vi "Consumer.vi"(8 "error in (no error)":errorcluster, 9 "Data":variant, 10 "Case ID":string, 11 "uService Template in":refnum<class "DAQ Manager.lvclass">) -> (0 "error out":errorcluster, 3 "uService Template out":refnum<class "DAQ Manager.lvclass">)   [LabVIEW 2020, in "TALOS.lvlib" / "DAQ Manager.lvlib" / "DAQ Manager.lvclass"]
uses:
  DAQ Manager.lvclass
  C:/LabVIEW Code/TALOS/talos/Father of all uServices/Father of all uServices/Father of all uServices.lvclass
  DAQ Manager Consumer Case Selector.ctl
  Father of all uServices/Father of all uServices/Father of all uServices.lvclass/Father of all uServices.ctl
  Ancestor/Ancestor/Ancestor.lvclass/Ancestor.ctl
  Guardian/Guardian/Requests.ctl
  Guardian/Guardian Messages/Requests from uServices Msg/Requests from uServices Msg.lvclass/Requests from uServices Msg.ctl
  Guardian/Guardian Messages/Message to uService Msg/Message to uService Msg.lvclass/Message to uService Msg.ctl
  Interfaces/DAQ Control/Metadata.ctl
  Guardian/Guardian Messages/Requests from uServices Msg/Send Requests from uServices.vi
  Support VIs/Generate Error.vi
  Father of all uServices/Father of all uServices/Children Methods/Message to uService.vi
  FGV/Error Memory/Get Error Description.vi
  Support VIs/Get PC name.vi
  Ancestor/Ancestor/Read ID.vi
  Support VIs/Get Class Name.vi
  <vilib>/Utility/error.llb/Clear Errors.vi
  Guardian/Guardian Messages/Message to uService Msg/Send Message to uService.vi
  FGV/Error Memory/Error Memory Core.vi
  <vilib>/AdvancedString/Delimited String to 1D String Array.vi
  Support VIs/Circus Root Path.vi
  FGV/Error Memory/Error Crt Lvl checker.vi
  FGV/Error Memory/Error Memory Core.vi/40c8088d-b597-4017-91af-faa98e00292e.vi
  FGV/Error Memory/Error Memory Core.vi/d4a3ab98-063c-4e44-b43d-fbdcfe6c2be2.vi
  Father of all uServices/Father of all uServices/Father of all uServices.lvclass
  C:/LabVIEW Code/TALOS/builds/Actor Framework PPL/Actor Framework.lvlibp/1abvi3w/vi.lib/ActorFramework/Actor/Actor.lvclass
  Support VIs/Global Memory.vi
  <vilib>/Utility/LVClass/Get LV Class Name.vi
  Support VIs/Is in Packed Library.vi
  Support VIs/TALOS Root path.vi
  Support VIs/Read CSV worksheet.vi
  Support VIs/Global Constants.vi
  <vilib>/Utility/error.llb/General Error Handler.vi
  Support VIs/Error Log.vi
  builds/Actor Framework PPL/Actor Framework.lvlibp/1abvi3w/vi.lib/ActorFramework/Actor/Read Caller Enqueuer.vi
  builds/Actor Framework PPL/Actor Framework.lvlibp/1abvi3w/vi.lib/ActorFramework/Message Enqueuer/Enqueue.vi
  Ancestor/Ancestor/Ancestor.lvclass
  <vilib>/Comparison/Equal/Equal Functor/Equal Functor.lvclass
  Guardian/Guardian Messages/Requests from uServices Msg/Requests from uServices Msg.lvclass
  Guardian/Guardian Messages/Message to uService Msg/Message to uService Msg.lvclass
  Guardian/Guardian/Guardian.lvclass
  Interfaces/DAQ Control/DAQ Control.lvclass
  TALOS.lvlib
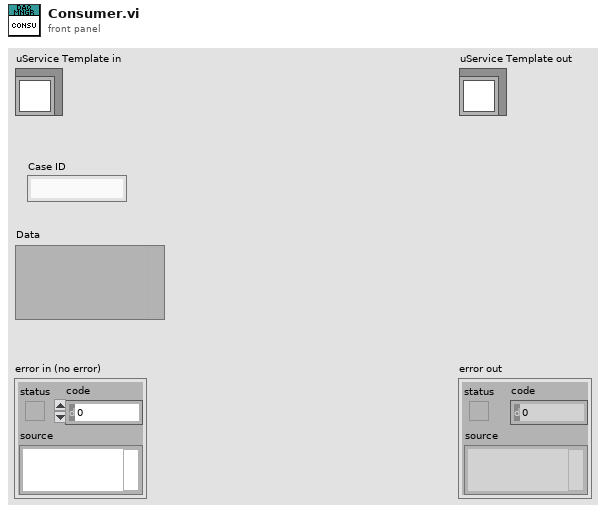
[diagram p1: front panel]
types:
  T1 = typedef "TALOS.lvlib/DAQ Manager.lvlib/DAQ Manager.lvclass/DAQ Manager Consumer Case Selector.ctl" = enum16{"Start Run", "Get Run Status", "Stop Run", "Send metadata to DAQ", "Test send DAQ"}
  T2 = typedef "TALOS.lvlib/Guardian.lvlib/Guardian.lvclass/Requests.ctl" = enum16{"Ready to Launch", "Start RUN", "Stop RUN", "Update DAQ Params", "Update Error Listbox", "Update Run Status", "Update Kasli Log", "Run Stopped with Errors", "Switch uS View"}
  T3 = typedef "TALOS.lvlib/Interfaces.lvlib/DAQ Control.lvclass/Metadata.ctl" = cluster{"Key":string, "Value":string}
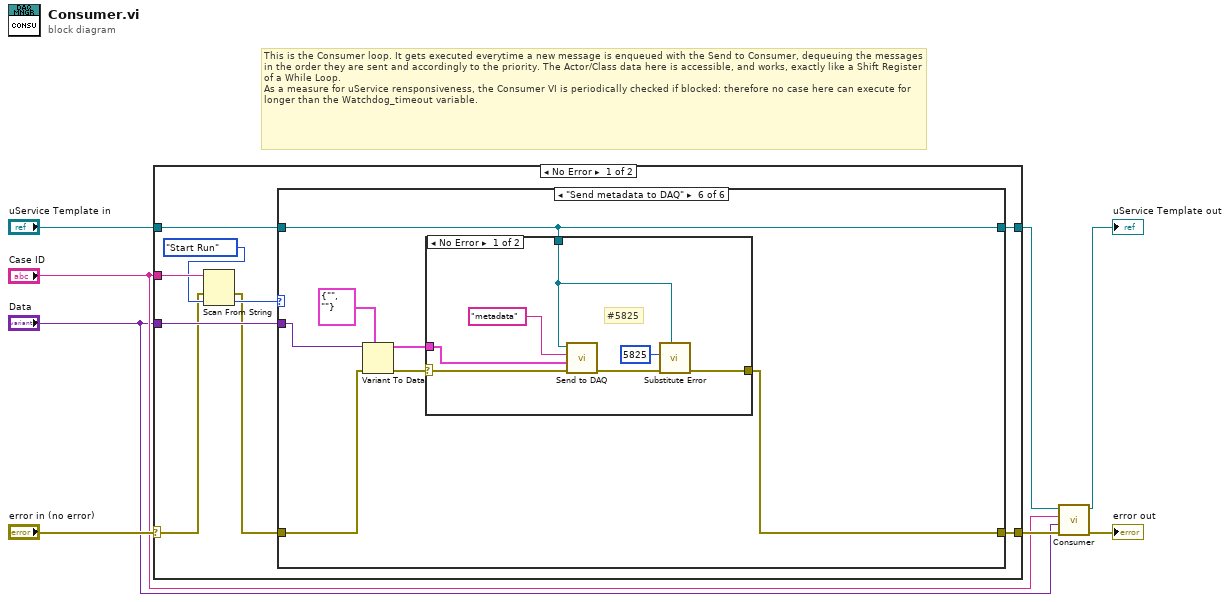
[diagram p0: block diagram]
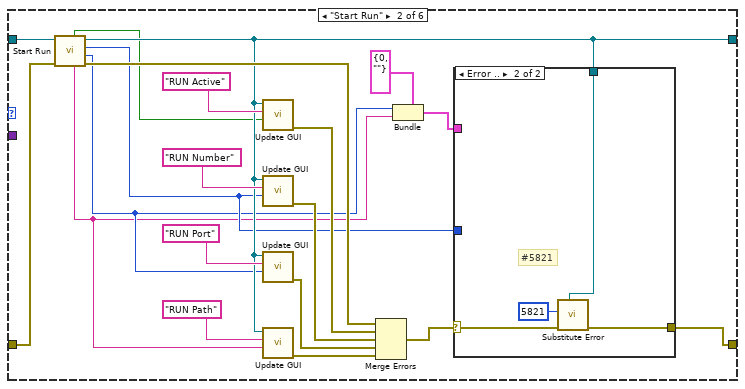
[diagram p3: hidden frame]
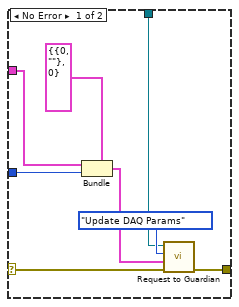
[diagram p4: hidden frame]
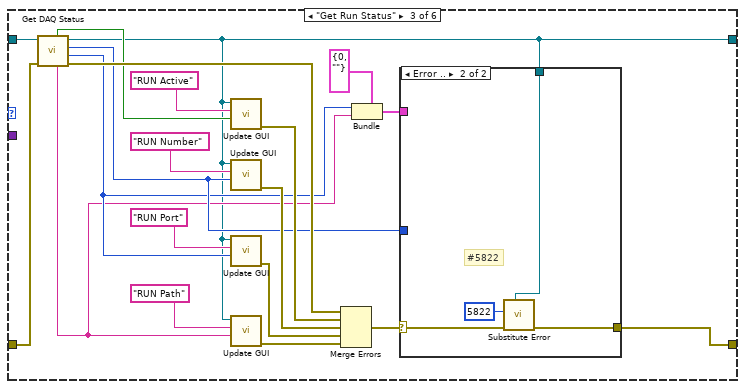
[diagram p5: hidden frame]
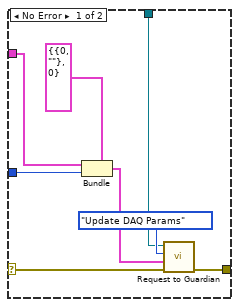
[diagram p6: hidden frame]
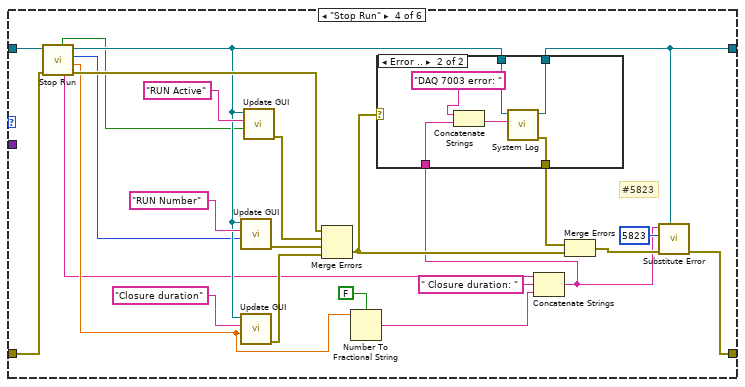
[diagram p7: hidden frame]
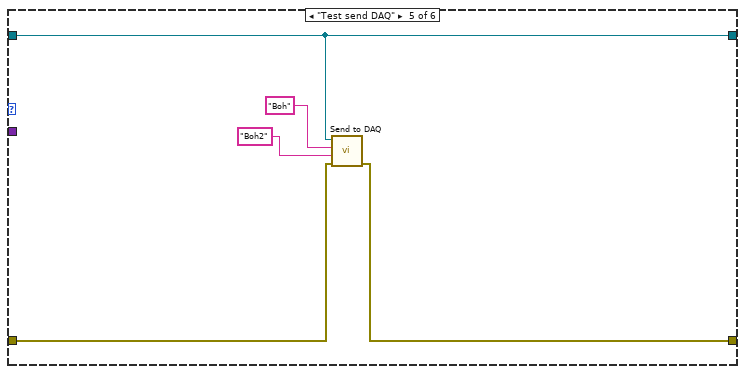
[diagram p9: hidden frame]
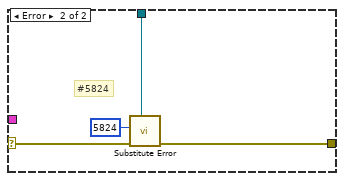
[diagram p10: hidden frame]
diagram:
  # "This is the Consumer loop. It gets executed everytime a new message is enqueued with the Send to Consumer, dequeuing the messages in the order they are sent and accordingly to the priority. The Actor/Class data here is accessible, and works, exactly like a Shift Register of a While Loop. \nAs a measure for uService rensponsiveness, the Consumer VI is periodically checked if blocked: therefore no case here can execute for longer than the Watchdog_timeout variable."
  n1 = case shown="No Error" "error in (no error)" {
    selector: "error in (no error)" -> [w10 w139]
    tunnel: [w16 w140] -> w4
    tunnel: "uService Template in" -> [w17 w140]
    tunnel: [w14 w139] -> w8
    tunnel: "Case ID" -> [w13 _]
    tunnel: "Data" -> [w15 _]
    frame No Error {
      n2 = Scan From String(input string=w13, error in=w10, default 1=DAQ_Manager_Consumer_Case_Selector."Start Run" ("Consumer Case Selector")) -> (error out=w9:errorcluster, output 1=w11:T1)  [unwired: 2 in, 2 out]
      n3 = case shown="\"Send metadata to DAQ\"" w11 {
        tunnel: w17 -> [w19 w26 w58 w90 w120 w123]
        tunnel: [w19 w25 w52 w94 w120 w123] -> w16
        tunnel: w15 -> [_ _ _ _ _ w124]
        tunnel: [w18 w28 w59 w102 w116 w121] -> w14
        tunnel: w9 -> [w18 w20 w57 w88 w117 w122]
        frame Default {
        }
        frame "Start Run" {
          n4 = call-dynamic "Start Run.vi"("error in (no error)"=w20, "DAQ Manager in"=w26) -> ("error out"=w39:errorcluster, "TCP Port Number"=w22:u32, "Run Number"=w23:u32, "DAQ Manager out"=w25:refnum<class "DAQ Manager.lvclass">, "Data storage path"=w21:string, "Run Active?"=w24:bool)  [unwired: 4 in]
          n5 = call "Update GUI.vi"("Data"=w24, "GUI Item Name"="RUN Active", "uService Template in"=w25) -> ("error out"=w33:errorcluster)  [unwired: 7 in, 1 out]
          n6 = call "Update GUI.vi"("Data"=w23, "GUI Item Name"="RUN Number", "uService Template in"=w25) -> ("error out"=w32:errorcluster)  [unwired: 7 in, 1 out]
          n7 = call "Update GUI.vi"("Data"=w22, "GUI Item Name"="RUN Port", "uService Template in"=w25) -> ("error out"=w31:errorcluster)  [unwired: 7 in, 1 out]
          n8 = call "Update GUI.vi"("Data"=w21, "GUI Item Name"="RUN Path", "uService Template in"=w25) -> ("error out"=w30:errorcluster)  [unwired: 7 in, 1 out]
          n9 = Merge Errors(w39, w33, w32, w31, w30) -> (w29:errorcluster)
          n10 = Bundle(cluster=cluster{u16, string} {0, ""}, w22, w21) -> (w27:cluster{u16, string})
          n11 = case shown="Error .." w29 {
            selector: w29 -> [w46 w51]
            tunnel: [w45 w50] -> w28
            tunnel: w25 -> [w44 w49]
            tunnel: w27 -> [w42 _]
            tunnel: w23 -> [w41 _]
            frame No Error {
              n12 = Bundle(cluster=cluster{cluster{u16, string}, i32} {{0, ""}, 0}, w42, w41) -> (w40:cluster{cluster{u16, string}, i32})
              n13 = call "Request to Guardian.vi"("error in (no error)"=w46, "Data"=w40, "Requests"=Requests."Update DAQ Params", "Father of all uServices in"=w44) -> ("error out"=w45:errorcluster)  [unwired: 6 in, 1 out]
            }
            frame Error {
              # "#5821"
              n14 = call "Substitute Error.vi"("LabVIEW Object"=w49, "error in (no error)"=w51, "Error Code"=5821) -> ("error out"=w50:errorcluster)  [unwired: 8 in]
            }
          }
        }
        frame "Get Run Status" {
          n15 = call-dynamic "Get DAQ Status.vi"("error in (no error)"=w57, "DAQ Manager in"=w58) -> ("error out"=w71:errorcluster, "TCP Port Number"=w54:u32, "Run Number"=w55:u32, "DAQ Manager out"=w52:refnum<class "DAQ Manager.lvclass">, "Data storage path"=w53:string, "Run Active?"=w56:bool)  [unwired: 4 in]
          n16 = call "Update GUI.vi"("Data"=w56, "GUI Item Name"="RUN Active", "uService Template in"=w52) -> ("error out"=w65:errorcluster)  [unwired: 7 in, 1 out]
          n17 = call "Update GUI.vi"("Data"=w55, "GUI Item Name"="RUN Number", "uService Template in"=w52) -> ("error out"=w64:errorcluster)  [unwired: 7 in, 1 out]
          n18 = call "Update GUI.vi"("Data"=w54, "GUI Item Name"="RUN Port", "uService Template in"=w52) -> ("error out"=w63:errorcluster)  [unwired: 7 in, 1 out]
          n19 = call "Update GUI.vi"("Data"=w53, "GUI Item Name"="RUN Path", "uService Template in"=w52) -> ("error out"=w62:errorcluster)  [unwired: 7 in, 1 out]
          n20 = Merge Errors(w71, w65, w64, w63, w62) -> (w61:errorcluster)
          n21 = Bundle(cluster=cluster{u16, string} {0, ""}, w54, w53) -> (w60:cluster{u16, string})
          n22 = case shown="Error .." w61 {
            selector: w61 -> [w78 w83]
            tunnel: [w77 w82] -> w59
            tunnel: w52 -> [w76 w81]
            tunnel: w60 -> [w74 _]
            tunnel: w55 -> [w73 _]
            frame No Error {
              n23 = Bundle(cluster=cluster{cluster{u16, string}, i32} {{0, ""}, 0}, w74, w73) -> (w72:cluster{cluster{u16, string}, i32})
              n24 = call "Request to Guardian.vi"("error in (no error)"=w78, "Data"=w72, "Requests"=Requests."Update DAQ Params", "Father of all uServices in"=w76) -> ("error out"=w77:errorcluster)  [unwired: 6 in, 1 out]
            }
            frame Error {
              # "#5822"
              n25 = call "Substitute Error.vi"("LabVIEW Object"=w81, "error in (no error)"=w83, "Error Code"=5822) -> ("error out"=w82:errorcluster)  [unwired: 8 in]
            }
          }
        }
        frame "Stop Run" {
          # "#5823"
          n26 = call-dynamic "Stop Run.vi"("error in (no error)"=w88, "DAQ Manager in"=w90) -> ("error out"=w107:errorcluster, "Closure duration"=w85:dbl, "Run Number"=w86:u32, "DAQ Manager out"=w89:refnum<class "DAQ Manager.lvclass">, "Comment"=w84:string, "Run Active?"=w87:bool)  [unwired: 4 in]
          n27 = call "Update GUI.vi"("Data"=w86, "GUI Item Name"="RUN Number", "uService Template in"=w89) -> ("error out"=w103:errorcluster)  [unwired: 7 in, 1 out]
          n28 = call "Update GUI.vi"("Data"=w85, "GUI Item Name"="Closure duration", "uService Template in"=w89) -> ("error out"=w99:errorcluster)  [unwired: 7 in, 1 out]
          n29 = call "Update GUI.vi"("Data"=w87, "GUI Item Name"="RUN Active", "uService Template in"=w89) -> ("error out"=w105:errorcluster)  [unwired: 7 in, 1 out]
          n30 = Merge Errors(w107, w105, w103, w99) -> (w95:errorcluster)
          n31 = Number To Fractional String(use system decimal point (T)=FALSE, number=w85) -> (F-format string=w97:string)  [unwired: 2 in]
          n32 = Concatenate Strings(w84, " Closure duration: " ("string"), w97) -> (w91:string)
          n33 = case shown="Error .." w95 {
            selector: w95 -> [w108 _]
            tunnel: w89 -> [w109 w115]
            tunnel: [w109 w114] -> w94
            tunnel: [w108 w113] -> w92
            tunnel: w91 -> [_ w111]
            frame No Error {
            }
            frame Error {
              n34 = Concatenate Strings("DAQ 7003 error: ", w111) -> (w110:string)
              n35 = call "System Log.vi"("Text to log"=w110, "uService Template in"=w115) -> ("error out"=w113:errorcluster, "uService Template out"=w114:refnum<class "DAQ Manager.lvclass">)  [unwired: 8 in]
            }
          }
          n36 = Merge Errors(w92, w95) -> (w93:errorcluster)
          n37 = call "Substitute Error.vi"("LabVIEW Object"=w94, "error in (no error)"=w93, "Error Code"=5823, "Optional String"=w91) -> ("error out"=w102:errorcluster)  [unwired: 7 in]
        }
        frame "Test send DAQ" {
          n38 = call "Send to DAQ.vi"("error in (no error)"=w117, "Data"="Boh2" ("Data Name"), "Data Name"="Boh", "Father of all uServices in"=w120) -> ("error out"=w116:errorcluster)  [unwired: 6 in, 1 out]
        }
        frame "Send metadata to DAQ" {
          n39 = Variant To Data(error in=w122, type=T3 {"Key"="", "Value"=""}, Variant=w124) -> (data=w125:T3, error out=w126:errorcluster)
          n40 = case shown="No Error" w126 {
            selector: w126 -> [w129 w136]
            tunnel: [w131 w135] -> w121
            tunnel: w123 -> [w132 w137]
            tunnel: w125 -> [w130 _]
            frame No Error {
              # "#5825"
              n41 = call "Send to DAQ.vi"("error in (no error)"=w129, "Data"=w130, "Data Name"="metadata", "Father of all uServices in"=w132) -> ("error out"=w128:errorcluster)  [unwired: 6 in, 1 out]
              n42 = call "Substitute Error.vi"("LabVIEW Object"=w132, "error in (no error)"=w128, "Error Code"=5825) -> ("error out"=w131:errorcluster)  [unwired: 8 in]
            }
            frame Error {
              # "#5824"
              n43 = call "Substitute Error.vi"("LabVIEW Object"=w137, "error in (no error)"=w136, "Error Code"=5824) -> ("error out"=w135:errorcluster)  [unwired: 8 in]
            }
          }
        }
      }
    }
    frame Error {
    }
  }
  n44 = call-parent "Consumer.vi"("error in (no error)"=w8, "Data"="Data", "Case ID"="Case ID", "uService Template in"=w4) -> ("error out"=→"error out":errorcluster, "uService Template out"=→"uService Template out":refnum<class "DAQ Manager.lvclass">)  [unwired: 6 in]
